vi "save_excel.vi"(10 "data in":string[][](array[string]), 11 "Path":path) -> ()   [LabVIEW 2017]
uses:
  <vilib>/addons/_office/excel.llb/Excel Easy Table (str).vi
  <vilib>/Utility/NIReport.llb/NI_report.lvclass
  <vilib>/addons/_office/NI_ReportGenerationToolkit.lvlib
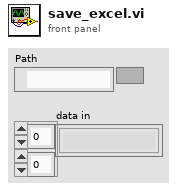
[diagram p1: front panel]
types:
  T1 = enum16{"Standard Report", "HTML", "Word", "Excel"}
  T2 = enum16{"maximized", "minimized", "normal", "no change"}
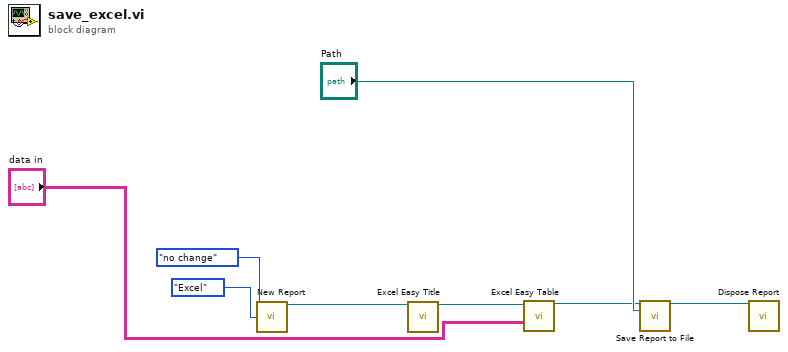
[diagram p0: block diagram]
diagram:
  n1 = call <vilib>:"New Report.vi"("window state (normal)"=T2."no change", "report type"=T1."Excel") -> ("report out"=w4:refnum<class "NI_report.lvclass">)  [unwired: 12 in, 1 out]
  n2 = call <vilib>:"Excel Easy Title.vi"("report in"=w4) -> ("report out"=w6:refnum<class "NI_report.lvclass">)  [unwired: 12 in, 2 out]
  n3 = call-poly <vilib>:"Excel Easy Table.vi"("report in"=w6, "text data"="data in") -> ("report out"=w7:refnum<class "NI_report.lvclass">)  [unwired: 9 in, 4 out]
  n4 = call-dynamic "Save Report to File.vi"("report in"=w7, "report file path"="Path") -> ("report out"=w1:refnum<class "NI_report.lvclass">)  [unwired: 12 in, 1 out]
  n5 = call-dynamic "Dispose Report.vi"("report in"=w1) -> ()  [unwired: 14 in, 1 out]
